vi "Digital Differential Analyzer.vi"(0 "x0":i32, 5 "y0":i32, 7 "x1":i32, 9 "y1":i32, 11 "error in (no error)":errorcluster) -> (4 "X coords":dbl[](array[numeric]), 6 "Y coords":dbl[](array[numeric]), 15 "error out":errorcluster)   [LabVIEW 2017]
doc: "To get the intermediate coords between the start point and end point in order to plot the desired linear."
panel:
  # "To get the intermediate coords between the start point and end point of a linear."
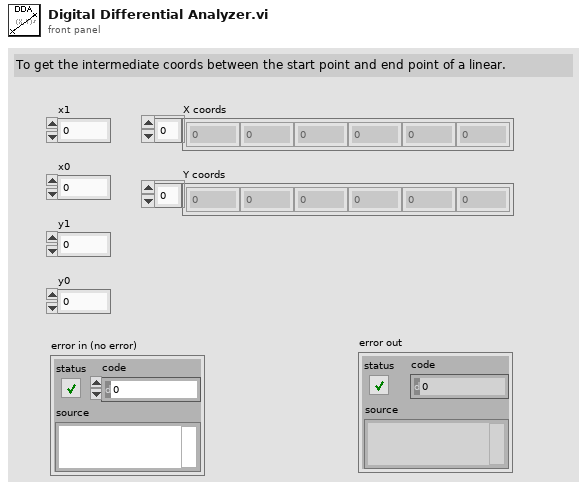
[diagram p1: front panel]
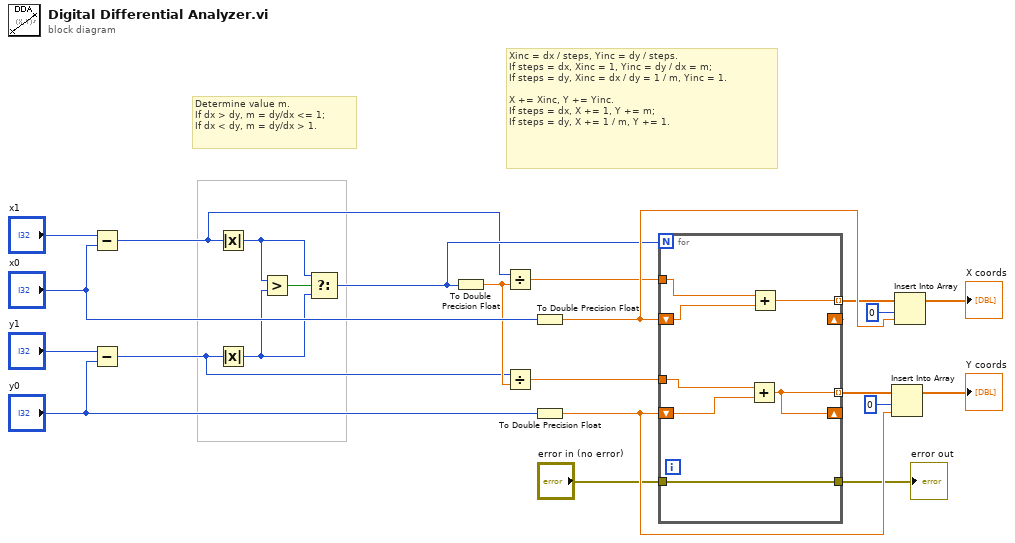
[diagram p0: block diagram]
diagram:
  # "Xinc = dx / steps, Yinc = dy / steps.\nIf steps = dx, Xinc = 1, Yinc = dy / dx = m;\nIf steps = dy, Xinc = dx / dy = 1 / m, Yinc = 1.\n\nX += Xinc, Y += Yinc.\nIf steps = dx, X += 1, Y += m;\nIf steps = dy, X += 1 / m, Y += 1."
  # "Determine value m.\nIf dx > dy, m = dy/dx <= 1;\nIf dx < dy, m = dy/dx > 1."
  n1 = Subtract(x="x1", y="x0") -> (x-y=w8:i32)
  n2 = Subtract(x="y1", y="y0") -> (x-y=w9:i32)
  n3 = Absolute Value(x=w8) -> (abs(x)=w6:i32)
  n4 = Absolute Value(x=w9) -> (abs(x)=w7:i32)
  n5 = Greater?(x=w6, y=w7) -> (0:w5:bool)
  n6 = Select(t=w6, s=w5, f=w7) -> (s? t:f=w11:i32)
  n7 = To Double Precision Float(number=w11) -> (double precision float=w10:dbl)
  n8 = Divide(x=w8, y=w10) -> (x/y=w12:dbl)
  n9 = Divide(x=w9, y=w10) -> (x/y=w13:dbl)
  n10 = To Double Precision Float(number="x0") -> (double precision float=w18:dbl)
  n11 = To Double Precision Float(number="y0") -> (double precision float=w21:dbl)
  n12 = for {
    N: w11 -> [_]
    tunnel: w12 -> [w30]
    tunnel: w13 -> [w27]
    shift-right: [w28] -> _
    shift-left: w18 -> [w29]
    shift-right: [w25] -> _
    shift-left: w21 -> [w26]
    tunnel: [w28] -> w17 mode=indexing
    tunnel: [w25] -> w19 mode=indexing
    tunnel: "error in (no error)" -> [w24]
    tunnel: [w24] -> w1
    n13 = Add(x=w27, y=w26) -> (x+y=w25:dbl)
    n14 = Add(x=w30, y=w29) -> (x+y=w28:dbl)
  }
  "error out" <- w1
  n15 = Insert Into Array(array=w19, index=0, new element=w21) -> (→"Y coords":dbl[])
  n16 = Insert Into Array(array=w17, index=0, new element=w18) -> (→"X coords":dbl[])
